vi "Populate Tree Items.vi"(8 "error in":errorcluster, 11 "EDS Viewer in":refnum<class "EDS Viewer.lvclass">) -> (0 "error out":errorcluster, 3 "EDS Viewer out":refnum<class "EDS Viewer.lvclass">)   [LabVIEW 2024, in "EDS Viewer.lvlib" / "EDS Viewer.lvclass"]
uses:
  EDS Viewer.lvclass
  EDS Viewer.lvclass/EDS Viewer.ctl
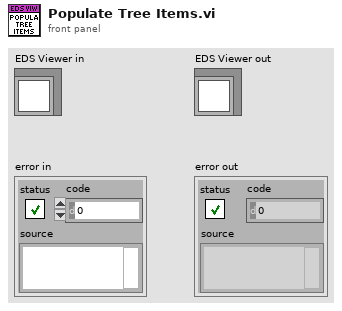
[diagram p1: front panel]
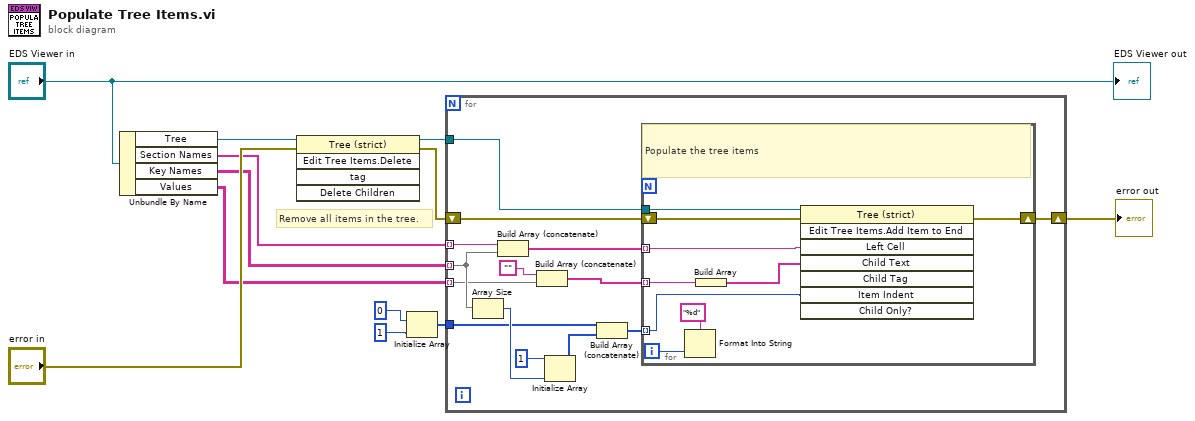
[diagram p0: block diagram]
diagram:
  # "Remove all items in the tree."
  n1 = Unbundle By Name("EDS Viewer in") -> ("Tree"=w11:refnum<vi>, "Section Names"=w7:string[], "Key Names"=w8:string[][], "Values"=w1:string[][])
  n2 = invoke on="Invoke Node" class="Tree (strict)" method="Edit Tree Items.Delete"(reference=w11, error in="error in") -> (reference out=w6:refnum<vi>, error out=w10:errorcluster)  [unwired: 3 in, 3 out]
  n3 = Initialize Array(0 ("element"), 1 ("dimension size")) -> (w2:i32[])
  n4 = for {
    tunnel: w8 -> [w20] mode=indexing
    tunnel: w7 -> [w25] mode=indexing
    tunnel: w6 -> [w24]
    shift-right: [w23] -> w5
    shift-left: w10 -> [w26]
    tunnel: w2 -> [w17]
    tunnel: w1 -> [w15] mode=indexing
    n5 = Array Size(array=w20) -> (size(s)=w19:i32)
    n6 = Build Array (concatenate)(w25, w20) -> (w22:string[])
    n7 = Build Array (concatenate)("", w15) -> (w14:string[])
    n8 = Initialize Array(1 ("dimension size"), w19) -> (w18:i32[])
    n9 = Build Array (concatenate)(w17, w18) -> (w16:i32[])
    n10 = for {
      tunnel: w22 -> [w34] mode=indexing
      shift-right: [w33] -> w23
      shift-left: w26 -> [w35]
      tunnel: w24 -> [w32]
      tunnel: w16 -> [w29] mode=indexing
      tunnel: w14 -> [w28] mode=indexing
      i -> [w31]
      # "Populate the tree items"
      n11 = Format Into String(format string="%d", w31) -> ()  [unwired: 2 in, 2 out]
      n12 = Build Array(w28) -> (w27:string[])
      n13 = invoke on="Invoke Node" class="Tree (strict)" method="Edit Tree Items.Add Item to End"(reference=w32, error in=w35, "Left Cell"=w34, "Child Text"=w27, "Item Indent"=w29) -> (error out=w33:errorcluster)  [unwired: 3 in, 7 out]
    }
  }
  "error out" <- w5
  "EDS Viewer out" <- "EDS Viewer in"
